vi "CMD_Harvest.vi"(1 "Line":string) -> (0 "Done":bool)   [LabVIEW 2018]
panel:
  in  "Parameters":i32[](array[numeric])=[1, 1, 1, 1]
  in  "Subcommands":string[](array[string])=["motor", "at", "for", "until"]
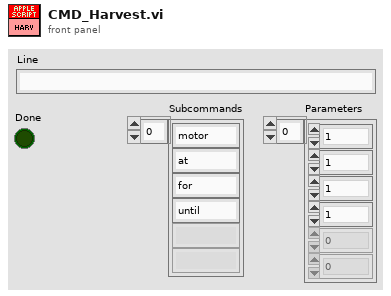
[diagram p1: front panel]
types:
  T1 = typedef "WPI_MotorControlDeviceRef.ctl" = cluster{"DeviceStatus":errorcluster, "Type":T2, "PWM":cluster{"PWM Channel":T3, "DeadBand":T4}, "CAN":cluster{"Device Number":u8, "SetOutput VI Ref":variant, "GetOutput VI Ref":variant, "Enable VI Ref":variant, "Disable VI Ref":variant, "Data":variant}, "Invert":bool, "DIO PWM":cluster{"PWM \"Enable\" Channel":T3, "DIOChannel":T5, "PWM Rate":dbl}}
  T2 = typedef "WPI_MotorControlType.ctl" = enum16{"PWM", "CAN", "DIO PWM"}
  T3 = typedef "FPGA_DIOPWMChannel.ctl" = enum8{"PWM 0", "PWM 1", "PWM 2", "PWM 3", "PWM 4", "PWM 5", "PWM 6", "PWM 7", "PWM 8", "PWM 9", "PWM MXP 0", "PWM MXP 1", "PWM MXP 2", "PWM MXP 3", "PWM MXP 4", "PWM MXP 5", "PWM MXP 6", "PWM MXP 7", "PWM MXP 8", "PWM MXP 9", "Invalid"}
  T4 = typedef "WPI_PWMDeadband.ctl" = cluster{"Name":string, "maxPositivePwm":i32, "minPositivePwm":i32, "centerPwm":i32, "maxNegativePwm":i32, "minNegativePwm":i32, "angularRange":u16}
  T5 = typedef "FPGA_DIOChannel.ctl" = enum8{"DIO 0", "DIO 1", "DIO 2", "DIO 3", "DIO 4", "DIO 5", "DIO 6", "DIO 7", "DIO 8", "DIO 9", "DIO MXP 0", "DIO MXP 1", "DIO MXP 2", "DIO MXP 3", "DIO MXP 4", "DIO MXP 5", "DIO MXP 6", "DIO MXP 7", "DIO MXP 8", "DIO MXP 9", "DIO MXP 10", "DIO MXP 11", "DIO MXP 12", "DIO MXP 13", "DIO MXP 14", "DIO MXP 15", "SPI Port CS1", "SPI Port CS2", "SPI Port CS3", "SPI Port MISO", "SPI Port MOSI", "Invalid"}
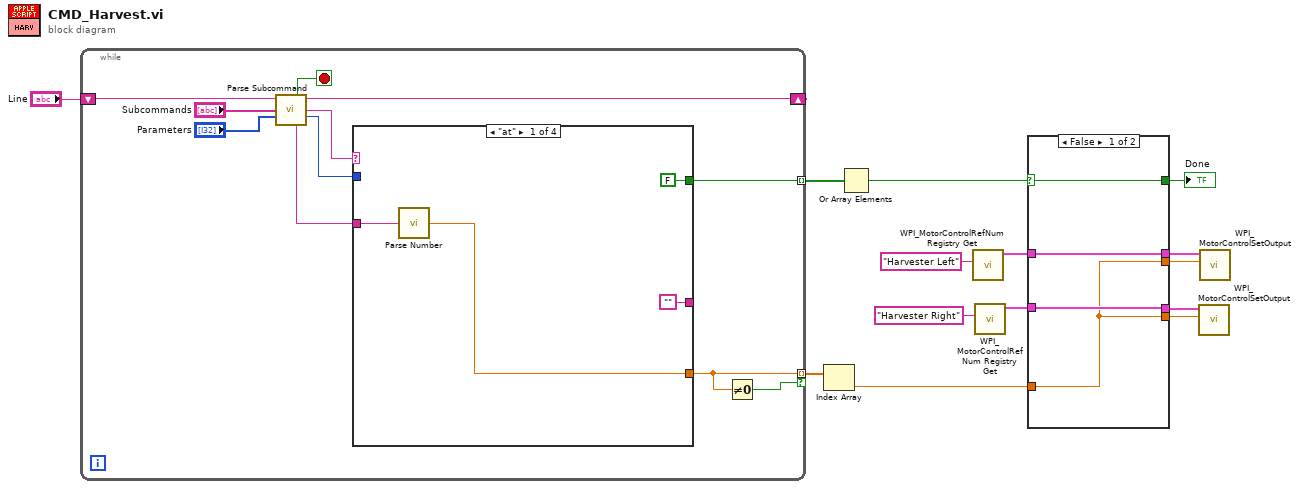
[diagram p0: block diagram]
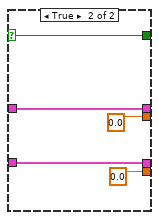
[diagram p2: hidden frame]
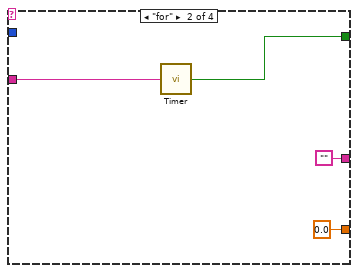
[diagram p3: hidden frame]
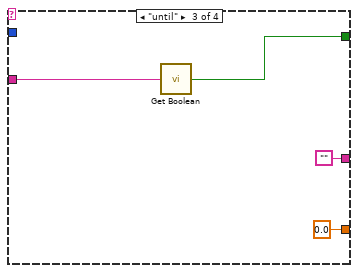
[diagram p4: hidden frame]
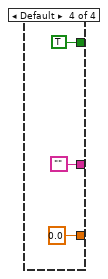
[diagram p5: hidden frame]
diagram:
  n1 = while {
    shift-right: [w22] -> _
    shift-left: "Line" -> [w25]
    tunnel: [w17] -> w13 mode=indexing
    tunnel: [w16] -> w12 mode=indexing if=w15
    stop <- w21 stop-if-true
    n2 = call "Parse Subcommand.vi"("Text In"=w25, "Subcommands"="Subcommands", "Parameters"="Parameters") -> ("Done"=w21:bool, "Text Out"=w22:string, "Subcommand"=w20:string, "# of Parameters"=w19:i32, "Parameter 1"=w18:string)  [unwired: 6 in, 2 out]
    n3 = case shown="\"at\"" w20 {
      tunnel: w19 -> [_ _ _ _]
      tunnel: w18 -> [w29 w33 w37 _]
      tunnel: [FALSE ("Value") w30 w34 TRUE ("Value")] -> w17
      tunnel: ["" "" "" ""] -> _
      tunnel: [w26 0.0 ("Number") 0.0 ("Number") 0.0 ("Number")] -> w16
      frame "at" {
        n4 = call "Parse Number.vi"("String"=w29) -> ("Number"=w26:dbl)
      }
      frame "for" {
        n5 = call "Timer.vi"("Seconds (string)"=w33) -> ("Done"=w30:bool)
      }
      frame "until" {
        n6 = call "Get Boolean.vi"("Name"=w37) -> ("Value"=w34:bool)
      }
      frame Default {
      }
    }
    n7 = Not Equal To 0?(x=w16) -> (x != 0?=w15:bool)
  }
  n8 = Index Array(array=w12) -> (element=w7:dbl)  [unwired: 1 in]
  n9 = Or Array Elements(Boolean array=w13) -> (logical OR=w11:bool)
  n10 = call <vilib>:"WPI_MotorControlRefNum Registry Get.vi"("refnum name"="Harvester Left") -> ("MotorControlDevRef"=w3:T1)  [unwired: 9 in, 1 out]
  n11 = call <vilib>:"WPI_MotorControlRefNum Registry Get.vi"("refnum name"="Harvester Right") -> ("MotorControlDevRef"=w9:T1)  [unwired: 9 in, 1 out]
  n12 = case shown="False" w11 {
    selector: w11 -> [w44 w49]
    tunnel: [w44 w49] -> w10
    tunnel: w9 -> [w43 w48]
    tunnel: [w43 w48] -> w8
    tunnel: w7 -> [w42 _]
    tunnel: [w42 0.0] -> w6
    tunnel: [w42 0.0] -> w1
    tunnel: w3 -> [w41 w45]
    tunnel: [w41 w45] -> w2
    frame False {
    }
    frame True {
    }
  }
  "Done" <- w10
  n13 = call <vilib>:"WPI_MotorControlSetOutput.vi"("Output"=w6, "MotorControlDevRef"=w8) -> ()  [unwired: 7 in, 3 out]
  n14 = call <vilib>:"WPI_MotorControlSetOutput.vi"("Output"=w1, "MotorControlDevRef"=w2) -> ()  [unwired: 7 in, 3 out]
